vi "P-P_Dis.vi"(3 "y2":dbl, 4 "y1":dbl, 5 "x2":dbl, 6 "x1":dbl) -> (0 "y":dbl, 1 "Dis":dbl, 2 "x":dbl)   [LabVIEW 2012]
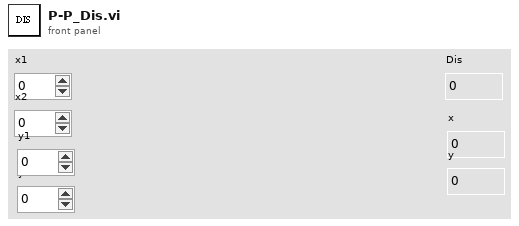
[diagram p1: front panel]
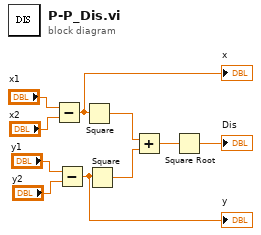
[diagram p0: block diagram]
diagram:
  n1 = Subtract(x="x1", y="x2") -> (x-y=w6:dbl)
  "x" <- w6
  n2 = Subtract(x="y1", y="y2") -> (x-y=w5:dbl)
  "y" <- w5
  n3 = Square(x=w6) -> (x^2=w4:dbl)
  n4 = Square(x=w5) -> (x^2=w3:dbl)
  n5 = Add(x=w4, y=w3) -> (x+y=w2:dbl)
  n6 = Square Root(x=w2) -> (sqrt(x)=→"Dis":dbl)
